vi "Initialize Attributes.vi"(8 "error in (no error)":errorcluster, 10 "Attribute Data":variant, 11 "DIMConnection in":refnum<class "DIMConnection.lvclass">) -> (0 "error out":errorcluster, 2 "Found?":bool, 3 "DIMConnection out":refnum<class "DIMConnection.lvclass">)   [LabVIEW 2016, in "CS++DIM.lvlib" / "DIMConnection.lvclass"]
doc: "Initialize object attribute.\n\nUnique resources should be allocated elsewhere!"
uses:
  DIMConnection.lvclass
  DIMConnection.lvclass/DIMConnection.ctl
  CSPP_Core/Classes/CS++ProcessVariables/PVConnection/PVConnection.lvclass
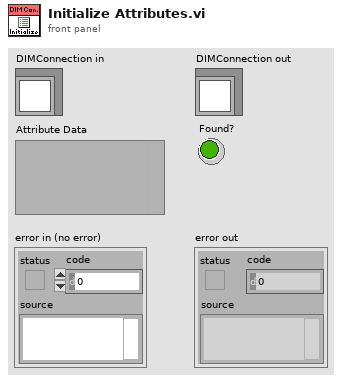
[diagram p1: front panel]
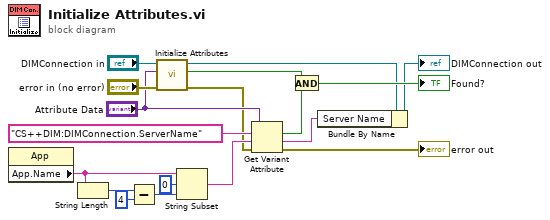
[diagram p0: block diagram]
diagram:
  n1 = property class="App"() -> ("App.Name"=w14:string)  [unwired: 2 in, 2 out]
  n2 = String Length(string=w14) -> (length=w12:i32)
  n3 = Subtract(x=w12, y=4) -> (x-y=w10:i32)
  n4 = call-parent "Initialize Attributes.vi"("error in (no error)"="error in (no error)", "Attribute Data"="Attribute Data", "PVConnection in"="DIMConnection in") -> ("error out"=w8:errorcluster, "Found?"=w5:bool, "PVConnection out"=w3:refnum<class "DIMConnection.lvclass">)  [unwired: 6 in]
  n5 = String Subset(string=w14, offset (0)=0, length (rest)=w10) -> (substring=w9:string)
  n6 = Get Variant Attribute(Variant="Attribute Data", name="CS++DIM:DIMConnection.ServerName", default value (empty Variant)=w9, error in=w8) -> (found=w6:bool, value=w1:string, error out=→"error out":errorcluster)  [unwired: 1 out]
  n7 = And(x=w5, y=w6) -> (x .and. y?=→"Found?":bool)
  n8 = Bundle By Name(cluster=w3, "Server Name"=w1) -> (→"DIMConnection out":refnum<class "DIMConnection.lvclass">)
